vi "UIdevelopment.vi"() -> ()   [LabVIEW 2020]
uses:
  <extravilib>/ChannelInstances/Tag-bool.lvlib
  <vilib>/ptbypt/NI_PtbyPt.lvlib
  <vilib>/express/express signal manip/GetorSetDDTAttributes/Set DDT Attributes/Set DDT Properties.xnode
  <vilib>/express/express shared/transition.llb/Dynamic To Waveform Array.vi
  <vilib>/express/express signal manip/GetorSetDDTAttributes/Set DDT Attributes/SetT0.vi
  <vilib>/express/express shared/transition.llb/Waveform Array To Dynamic.vi
panel:
  out "Current RMS [A]":dbl(knob) scale=0.0..20.0
  out "Power Output [W]":dbl(knob) scale=0.0..20.0
  out "Voltage RMS [V]":dbl(knob) scale=0.0..20.0
  in  "?":T1(tab)
  in  "File Path":path
  in  "Write Data to File":bool
  in  "Voltage Threshold":dbl
  out "dt":dbl
  in  "Sample rate":dbl=1000.0
  in  "Number of Samples":i32=5
  out "RPM 2":dbl
  out "Signal Frequency (Hz)":dbl format="%#_13g"
  in  "Number of teeth in gear":dbl
  in  "?":bool
  out "Hall sensor\n 2":dynamicdata(graph)
  out "Hall sensor":dynamicdata(graph)
  out "Voltage Sensor":dynamicdata(graph)
  out "Current Sensor":dynamicdata(graph)
  out "Omega [RPM]":dbl(knob) scale=0.0..2000.0
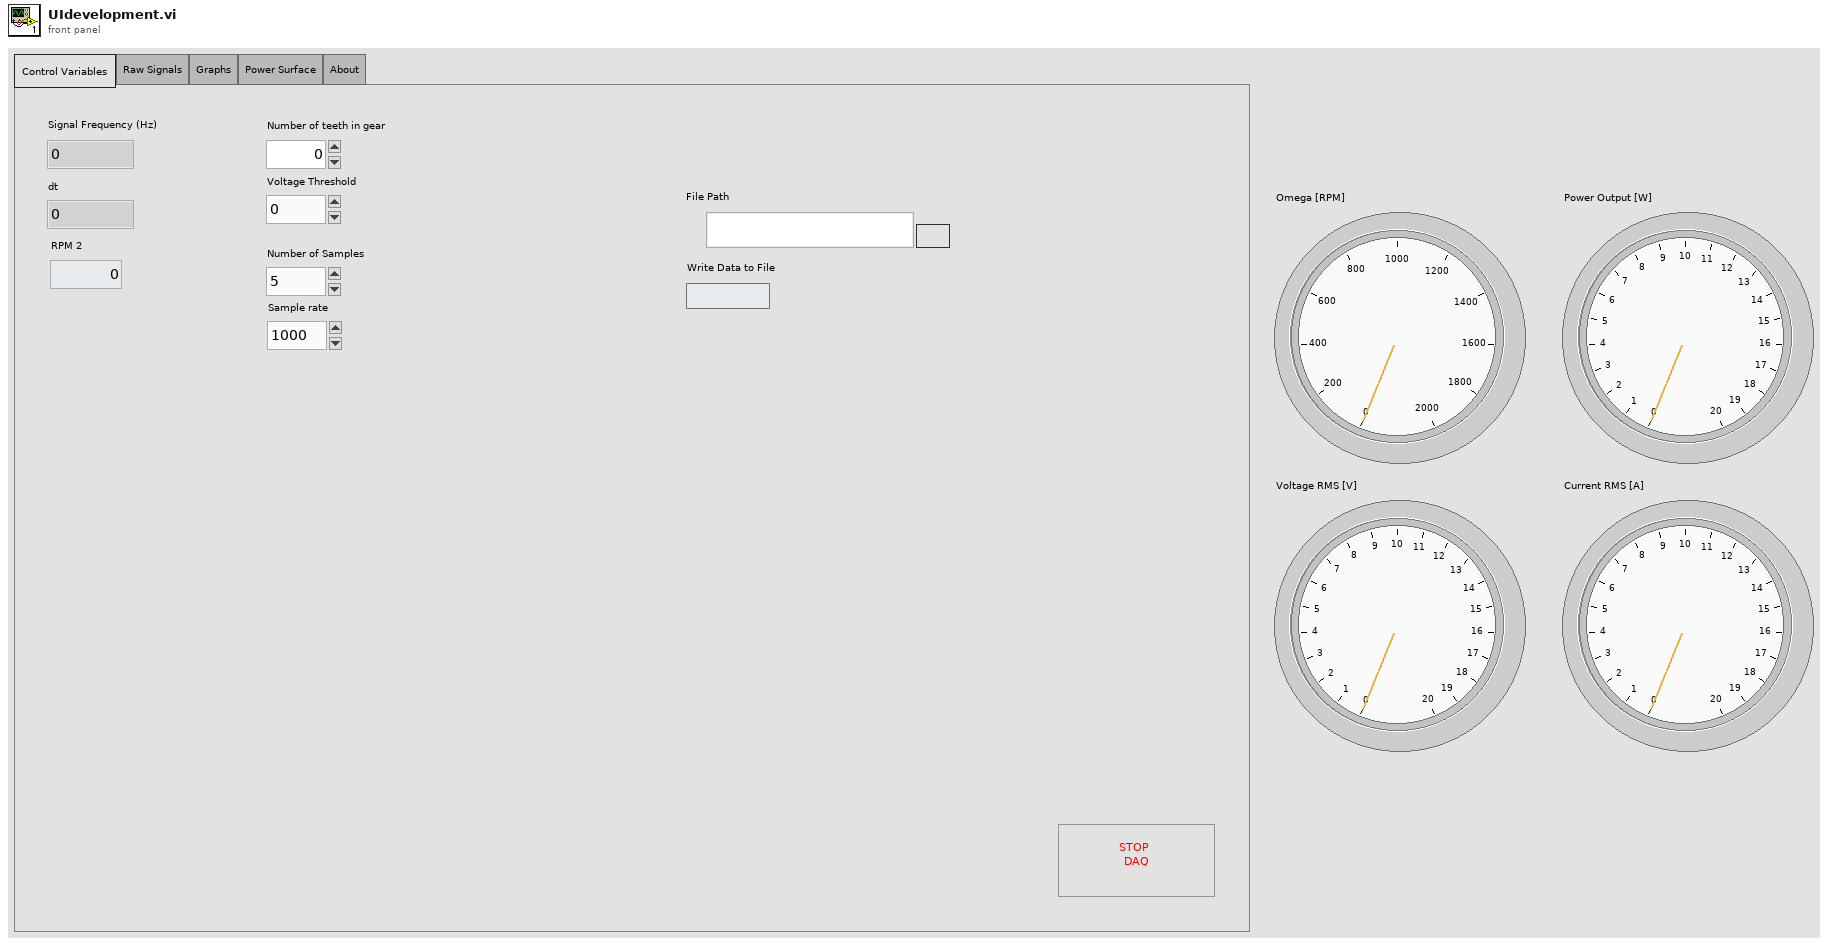
[diagram p1: front panel]
types:
  T1 = enum32{"Control Variables ", "Raw Signals", "Graphs", "Power Surface", "About"}
  T2 = typedef "Tag-bool.lvlib/))Channel.ctl" = refnum<queue>
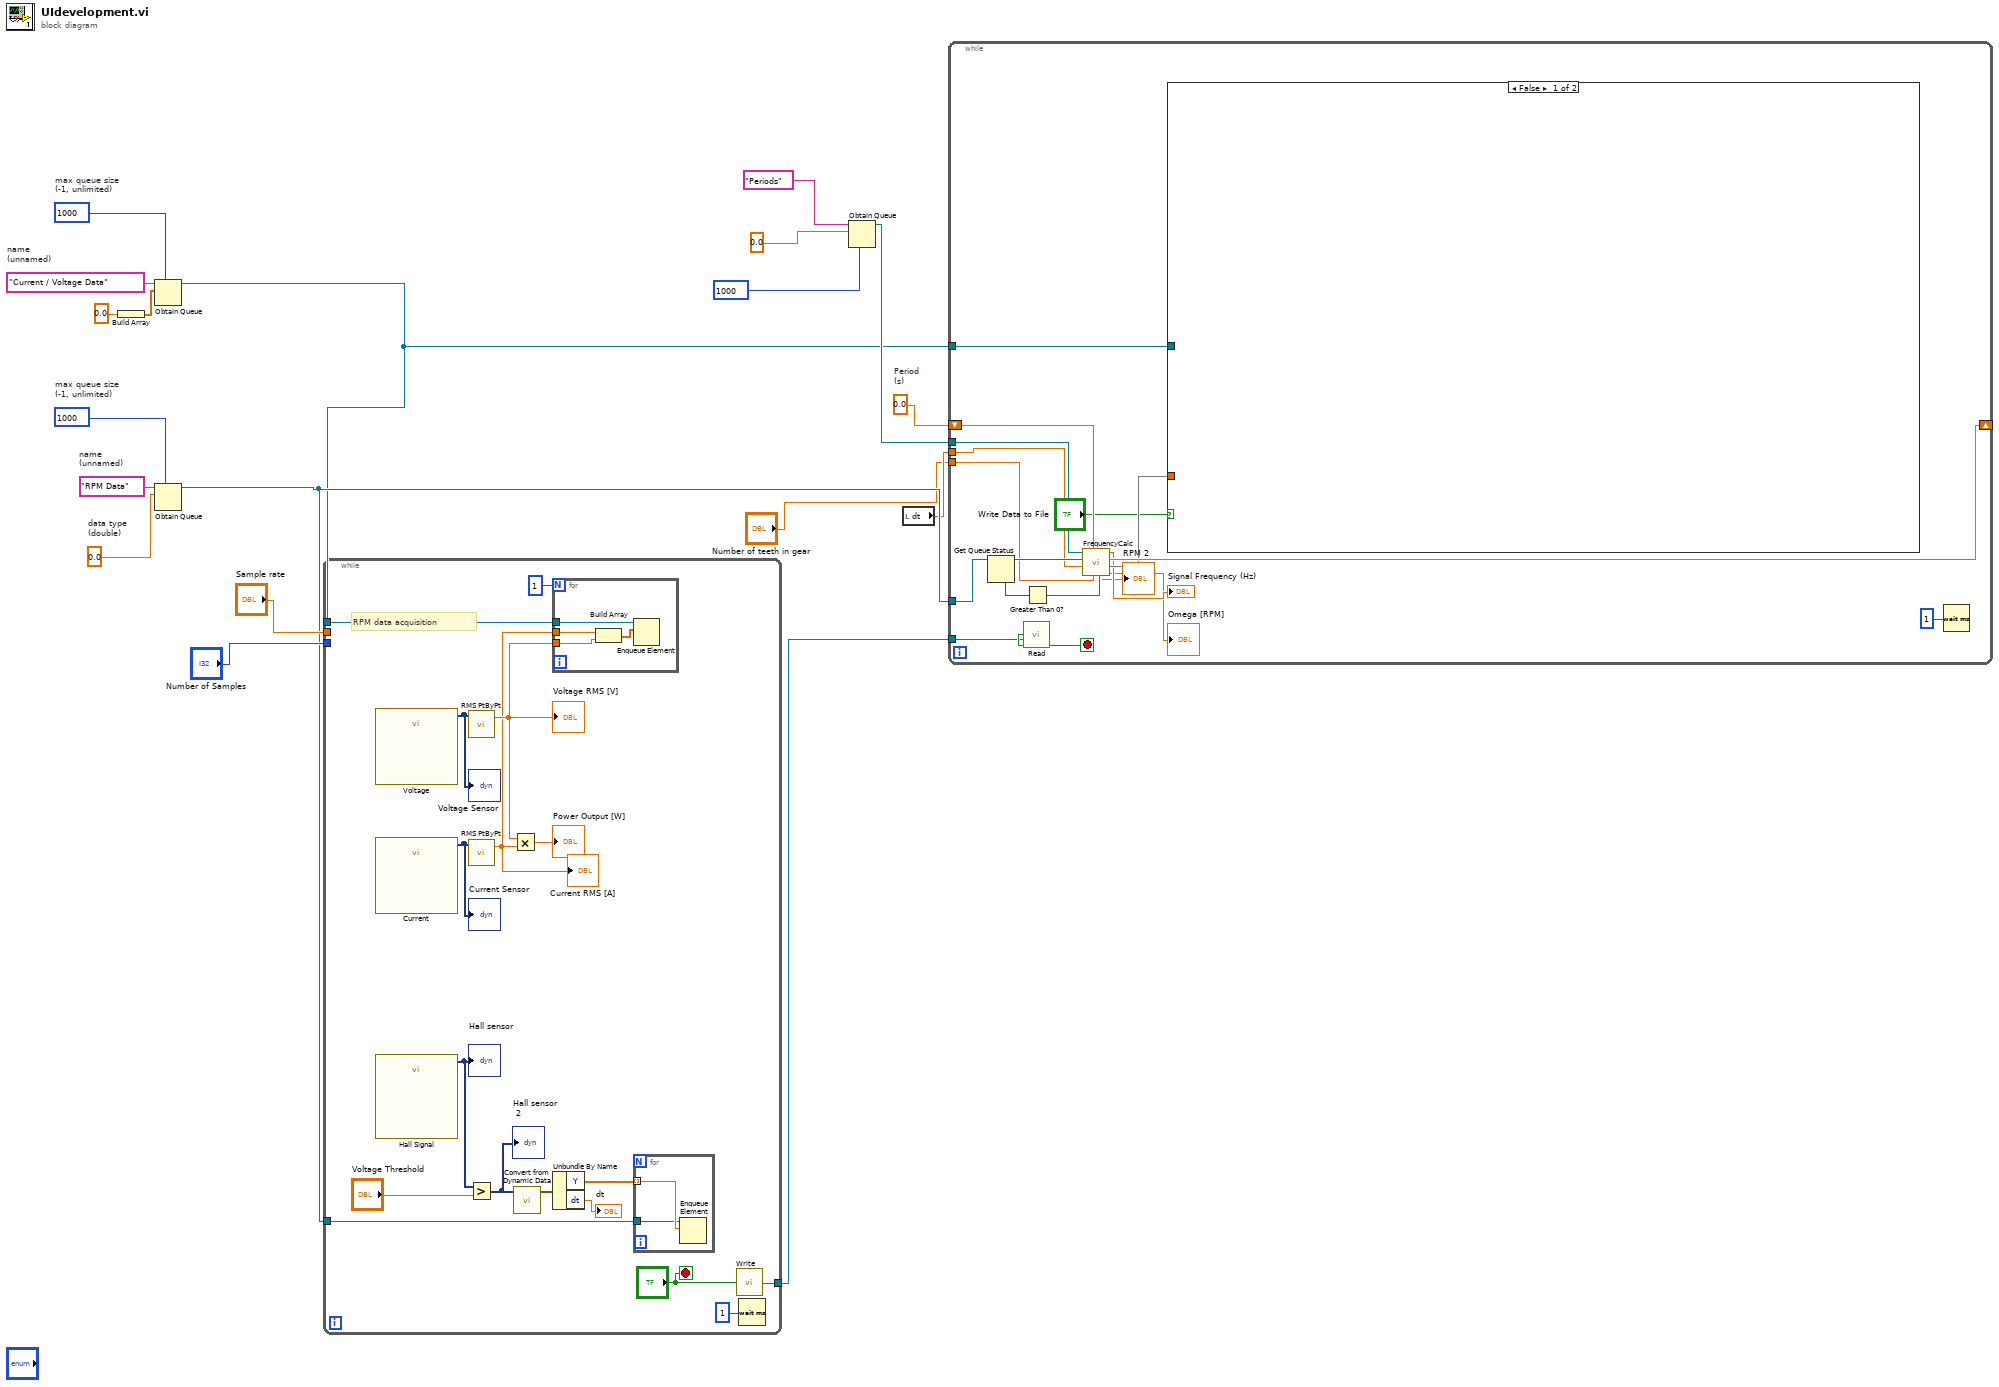
[diagram p0: block diagram]
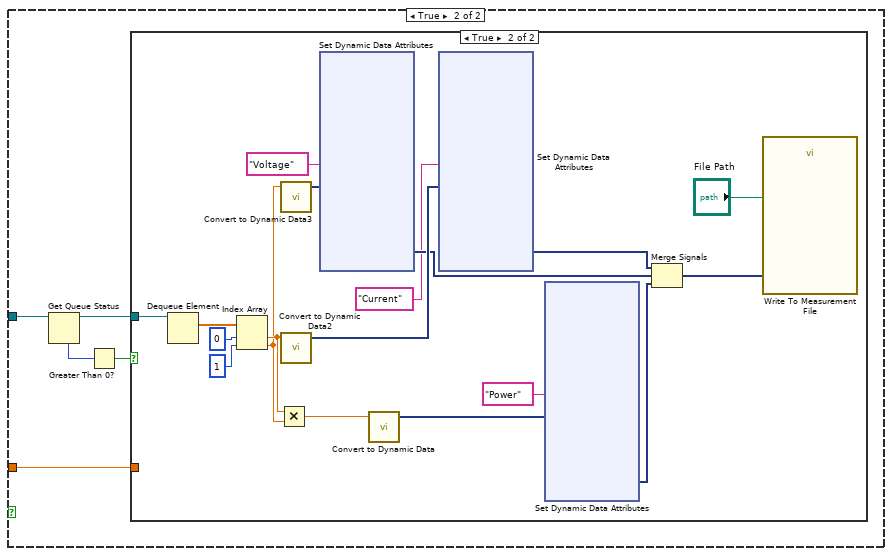
[diagram p2: hidden frame]
diagram:
  w4 = "Current / Voltage Data"  # name (unnamed)
  w5 = 1000  # max queue size (-1, unlimited)
  w9 = 0.0  # Period (s)
  w17 = 0.0  # data type (double)
  w18 = "RPM Data"  # name (unnamed)
  w19 = 1000  # max queue size (-1, unlimited)
  n1 = Build Array(0.0 ("element")) -> (w3:dbl[])
  n2 = Obtain Queue(max queue size (-1, unlimited)=w5, name (unnamed)=w4, element data type=w3) -> (queue out=w1:refnum<queue>)  [unwired: 2 in, 2 out]
  n3 = Obtain Queue(max queue size (-1, unlimited)=w19, name (unnamed)=w18, element data type=w17) -> (queue out=w10:refnum<queue>)  [unwired: 2 in, 2 out]
  n4 = while {
    tunnel: w10 -> [w34]
    tunnel: "Sample rate" -> [_]
    tunnel: "Number of Samples" -> [_]
    tunnel: [w29] -> w6
    tunnel: w1 -> [w26]
    stop <- "?" stop-if-true
    # "RPM data acquisition"
    n5 = call "Voltage"() -> ("Sine"=w27:dynamicdata)  [unwired: 14 in, 1 out]
    "Voltage Sensor" <- w27
    n6 = call "Current"() -> ("Sine"=w28:dynamicdata)  [unwired: 14 in, 1 out]
    "Current Sensor" <- w28
    n7 = call "Hall Signal"() -> ("Square"=w31:dynamicdata)  [unwired: 14 in, 1 out]
    "Hall sensor" <- w31
    n8 = call <vilib>:"RMS PtByPt.vi"("x"=w27) -> ("rms value"=w25:dbl)  [unwired: 3 in, 1 out]
    "Voltage RMS [V]" <- w25
    n9 = call <vilib>:"RMS PtByPt.vi"("x"=w28) -> ("rms value"=w24:dbl)  [unwired: 3 in, 1 out]
    "Current RMS [A]" <- w24
    n10 = Greater?(x=w31, y="Voltage Threshold") -> (0:w30:dynamicdata)
    "Hall sensor\n 2" <- w30
    n11 = Multiply(x=w25, y=w24) -> (x*y=→"Power Output [W]":dbl)
    n12 = call "Convert from Dynamic Data"("Dynamic Data Type"=w30) -> ("Waveform"=w36:waveform(dbl))  [unwired: 3 in]
    n13 = for {
      N: 1 -> [_]
      tunnel: w26 -> [w40]
      tunnel: w24 -> [w39]
      tunnel: w25 -> [w38]
      n14 = Build Array(w39, w38) -> (w37:dbl[])
      n15 = Enqueue Element(queue=w40, element=w37) -> ()  [unwired: 2 in, 3 out]
    }
    n16 = Unbundle By Name(w36) -> ("Y"=w35:dbl[], "dt"=→"dt":dbl)
    n17 = for {
      tunnel: w35 -> [w42] mode=indexing
      tunnel: w34 -> [w41]
      n18 = Enqueue Element(queue=w41, element=w42) -> ()  [unwired: 2 in, 3 out]
    }
    n19 = call <extravilib>:"Write.vi"("element"="?") -> ("channel"=w29:T2)  [unwired: 1 out]
    n20 = Wait (ms)(milliseconds to wait=u32 1) -> ()  [unwired: 1 out]
  }
  n21 = Obtain Queue(max queue size (-1, unlimited)=1000 ("max queue size\n(-1, unlimited)"), name (unnamed)="Periods" ("name\n(unnamed)"), element data type=0.0 ("data type\n(double)")) -> (queue out=w11:refnum<queue>)  [unwired: 2 in, 2 out]
  n22 = local read "dt"() -> (w8:dbl)
  n23 = while {
    tunnel: w10 -> [w59]
    tunnel: w11 -> [w56]
    shift-right: [w54] -> _
    shift-left: w9 -> [w55]
    tunnel: w8 -> [w50]
    tunnel: "Number of teeth in gear" -> [w53]
    tunnel: w6 -> [w51]
    tunnel: w1 -> [w49]
    stop <- w52 stop-if-true
    n24 = Get Queue Status(queue=w59) -> (queue out=w57:refnum<queue>, # elements in queue=w60:i32)  [unwired: 2 in, 6 out]
    n25 = call <extravilib>:"Read.vi"("channel"=w51) -> ("element"=w52:bool)  [unwired: 1 in, 1 out]
    n26 = Greater Than 0?(x=w60) -> (x > 0?=w58:bool)
    n27 = call "FrequencyCalc.vi"("Checkbox"=w58, "Number of teeth in gear"=w53, "Period\n(s) in"=w55, "dt"=w50, "queue in"=w57, "Queue in"=w56) -> ("Omega [RPM]"=→"Omega [RPM]":dbl, 1:w48, "Period\n(s) out"=w54:dbl, "Signal Frequency (Hz)"=→"Signal Frequency (Hz)":dbl, "RPM 2"=→"RPM 2":dbl)  [unwired: 1 in]
    n28 = case shown="False" "Write Data to File" {
      tunnel: w49 -> [_ w62]
      tunnel: w48 -> [_ w61]
      frame False {
      }
      frame True {
        n29 = Get Queue Status(queue=w62) -> (queue out=w63:refnum<queue>, # elements in queue=w65:i32)  [unwired: 2 in, 6 out]
        n30 = Greater Than 0?(x=w65) -> (x > 0?=w64:bool)
        n31 = case shown="True" w64 {
          tunnel: w63 -> [_ w80]
          tunnel: w61 -> [_ _]
          frame False {
          }
          frame True {
            n32 = Dequeue Element(queue=w80) -> (element=w83:dbl[])  [unwired: 2 in, 3 out]
            n33 = Index Array(array=w83, index #1=0 ("index"), index #2=1 ("index")) -> (element #1=w77:dbl, element #2=w76:dbl)
            n34 = Multiply(x=w77, y=w76) -> (x*y=w78:dbl)
            n35 = call "Convert to Dynamic Data3"("Double"=w76) -> ("Dynamic Data Type"=w74:dynamicdata)  [unwired: 3 in]
            n36 = call "Convert to Dynamic Data2"("Double"=w77) -> ("Dynamic Data Type"=w75:dynamicdata)  [unwired: 3 in]
            n37 = xnode "Set Dynamic Data Attributes"("Signal Name"="Voltage", "Signals In"=w74) -> ("Signals Out"=w71:dynamicdata)  [unwired: 2 in, 1 out]
            n38 = call "Convert to Dynamic Data"("Double"=w78) -> ("Dynamic Data Type"=w73:dynamicdata)  [unwired: 3 in]
            n39 = xnode "Set Dynamic Data Attributes"("Signal Name"="Current", "Signals In"=w75) -> ("Signals Out"=w72:dynamicdata)  [unwired: 2 in, 1 out]
            n40 = xnode "Set Dynamic Data Attributes"("Signal Name"="Power", "Signals In"=w73) -> ("Signals Out"=w70:dynamicdata)  [unwired: 2 in, 1 out]
            n41 = Merge Signals(w72, w71, w70) -> (w69:dynamicdata)
            n42 = call "Write To Measurement File"("Signals"=w69, "Filename"="File Path") -> ()  [unwired: 15 in, 3 out]
          }
        }
      }
    }
    n43 = Wait (ms)(milliseconds to wait=u32 1) -> ()  [unwired: 1 out]
  }
